vi "Error Query Channel.vi"(7 "Channel (0: SIM900)":i32(ring) items=["SIM900", "1", "2", "3", "4", "5", "6", "7", "8", "9", "A", "B", "C", "D"], 8 "error in (no error)":errorcluster, 11 "VISA resource name":refnum<visa-resource-name>) -> (0 "error out":errorcluster, 1 "Error Message":string, 2 "Error Code":i32, 3 "VISA resource name out":refnum<visa-resource-name>)   [LabVIEW 2019, in "Stanford Research SIM900 Series.lvlib"]
doc: "Preforme error query on the specified port or the SIM900."
uses:
  Stanford Research SIM900 Series.lvlib
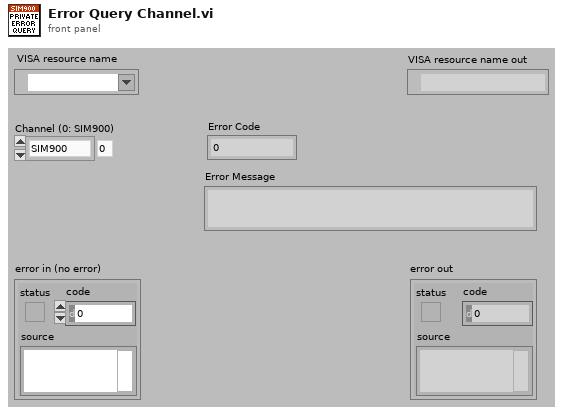
[diagram p1: front panel]
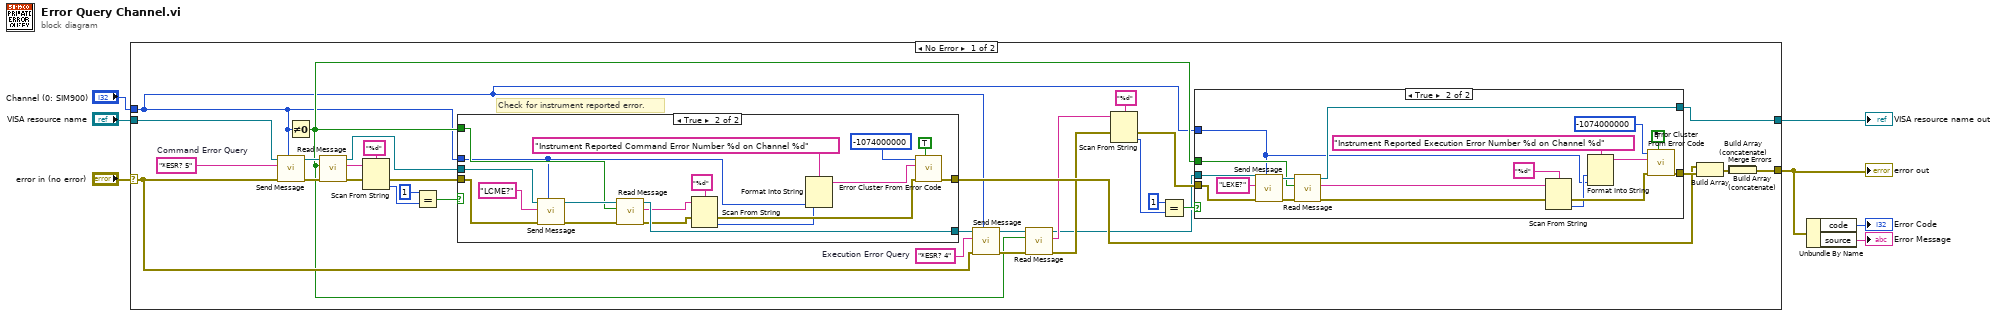
[diagram p0: block diagram]
diagram:
  n1 = case shown="No Error" "error in (no error)" {
    selector: "error in (no error)" -> [w25 w83]
    tunnel: [w39 w83] -> w3
    tunnel: [w30 w82] -> w4
    tunnel: "VISA resource name" -> [w29 w82]
    tunnel: "Channel (0: SIM900)" -> [w11 _]
    frame No Error {
      w12 = "*ESR? 4"  # Execution Error Query
      w13 = "*ESR? 5"  # Command Error Query
      # "Check for instrument reported error."
      n2 = call "Send Message.vi"("Channel (0: SIM900)"=w11, "error in (no error)"=w25, "Message (\"\")"=w13, "VISA resource name"=w29) -> ("error out"=w18:errorcluster, "VISA resource name out"=w19:refnum<visa-resource-name>)  [unwired: 6 in]
      n3 = Not Equal To 0?(x=w11) -> (x != 0?=w15:bool)
      n4 = call "Read Message.vi"("error in (no error)"=w18, "Enable Header Information (False)"=w15, "VISA resource name"=w19) -> ("error out"=w17:errorcluster, "Message"=w14:string, "VISA resource name out"=w16:refnum<visa-resource-name>)  [unwired: 6 in]
      n5 = Scan From String(format string="%d", input string=w14, error in=w17) -> (error out=w27:errorcluster, output 1=w36:i32)  [unwired: 2 in, 2 out]
      n6 = Equal?(x=1, y=w36) -> (x = y?=w35:bool)
      n7 = case shown="True" w35 {
        tunnel: w16 -> [w43 w58]
        tunnel: [w43 w48] -> w28
        tunnel: [w42 w57] -> w26
        tunnel: w27 -> [w42 w56]
        tunnel: w15 -> [_ w49]
        tunnel: w11 -> [_ w44]
        frame False {
        }
        frame True {
          n8 = call "Send Message.vi"("Channel (0: SIM900)"=w44, "error in (no error)"=w56, "Message (\"\")"="LCME?" ("write buffer"), "VISA resource name"=w58) -> ("error out"=w50:errorcluster, "VISA resource name out"=w51:refnum<visa-resource-name>)  [unwired: 6 in]
          n9 = call "Read Message.vi"("error in (no error)"=w50, "Enable Header Information (False)"=w49, "VISA resource name"=w51) -> ("error out"=w47:errorcluster, "Message"=w46:string, "VISA resource name out"=w48:refnum<visa-resource-name>)  [unwired: 6 in]
          n10 = Scan From String(format string="%d", input string=w46, error in=w47) -> (error out=w59:errorcluster, output 1=w54:i32)  [unwired: 2 in, 2 out]
          n11 = Format Into String(format string="Instrument Reported Command Error Number %d on Channel %d", w54, w44) -> (resulting string=w52:string)  [unwired: 2 in, 1 out]
          n12 = call <vilib>:"Error Cluster From Error Code.vi"("show call chain? (False)"=TRUE, "error in (no error)"=w59, "error message (\"\")"=w52, "error code (0)"=-1074000000) -> ("error out"=w57:errorcluster)  [unwired: 5 in]
        }
      }
      n13 = call "Send Message.vi"("Channel (0: SIM900)"=w11, "error in (no error)"=w25, "Message (\"\")"=w12, "VISA resource name"=w28) -> ("error out"=w23:errorcluster, "VISA resource name out"=w24:refnum<visa-resource-name>)  [unwired: 6 in]
      n14 = call "Read Message.vi"("error in (no error)"=w23, "Enable Header Information (False)"=w15, "VISA resource name"=w24) -> ("error out"=w21:errorcluster, "Message"=w22:string, "VISA resource name out"=w20:refnum<visa-resource-name>)  [unwired: 6 in]
      n15 = Scan From String(format string="%d", input string=w22, error in=w21) -> (error out=w37:errorcluster, output 1=w34:i32)  [unwired: 2 in, 2 out]
      n16 = Equal?(x=1, y=w34) -> (x = y?=w33:bool)
      n17 = case shown="True" w33 {
        tunnel: [w63 w79] -> w40
        tunnel: w37 -> [w63 w78]
        tunnel: w20 -> [w62 w77]
        tunnel: [w62 w69] -> w30
        tunnel: w15 -> [_ w66]
        tunnel: w11 -> [_ w64]
        frame False {
        }
        frame True {
          n18 = call "Send Message.vi"("Channel (0: SIM900)"=w64, "error in (no error)"=w78, "Message (\"\")"="LEXE?" ("write buffer"), "VISA resource name"=w77) -> ("error out"=w70:errorcluster, "VISA resource name out"=w71:refnum<visa-resource-name>)  [unwired: 6 in]
          n19 = call "Read Message.vi"("error in (no error)"=w70, "Enable Header Information (False)"=w66, "VISA resource name"=w71) -> ("error out"=w68:errorcluster, "Message"=w67:string, "VISA resource name out"=w69:refnum<visa-resource-name>)  [unwired: 6 in]
          n20 = Scan From String(format string="%d", input string=w67, error in=w68) -> (error out=w76:errorcluster, output 1=w74:i32)  [unwired: 2 in, 2 out]
          n21 = Format Into String(format string="Instrument Reported Execution Error Number %d on Channel %d", w74, w64) -> (resulting string=w73:string)  [unwired: 2 in, 1 out]
          n22 = call <vilib>:"Error Cluster From Error Code.vi"("show call chain? (False)"=TRUE, "error in (no error)"=w76, "error message (\"\")"=w73, "error code (0)"=-1074000000) -> ("error out"=w79:errorcluster)  [unwired: 5 in]
        }
      }
      n23 = Build Array(w26, w40) -> (w10:errorcluster[])
      n24 = Build Array (concatenate)(w10) -> (w9:errorcluster[])
      n25 = Build Array (concatenate)(w9) -> (w8:errorcluster[])
      n26 = Merge Errors(w8) -> (w39:errorcluster)
    }
    frame Error {
    }
  }
  "error out" <- w3
  "VISA resource name out" <- w4
  n27 = Unbundle By Name(w3) -> ("code"=→"Error Code":i32, "source"=→"Error Message":string)
